vi "io.command-builder.DI.vi"(8 "error in":errorcluster, 11 "IoConf in":T1={"ADDR"=0, "Label"="", "Type"=enum."DI", "Mode"=enum."RIO", "Value"="", "Tags"="", "calibration"=[]} {"calibration"."Y" format="%#.3f"; "calibration"."X" format="%#.3f"; "ADDR" format="%04d"}) -> (0 "error out":errorcluster, 2 "Generated Command":string)   [LabVIEW 2024]
uses:
  controls/IONode.ctl
  controls/type.address.ctl
  controls/enum.io.type.ctl
  controls/enum.io.mode.ctl
  controls/typeXyPoint.ctl
  controls/enum.io-rio.ctl
  variantCtrlNumber.vi
panel:
  in  "Value in":cluster{"value":u8, "timeoutSeconds":u16}
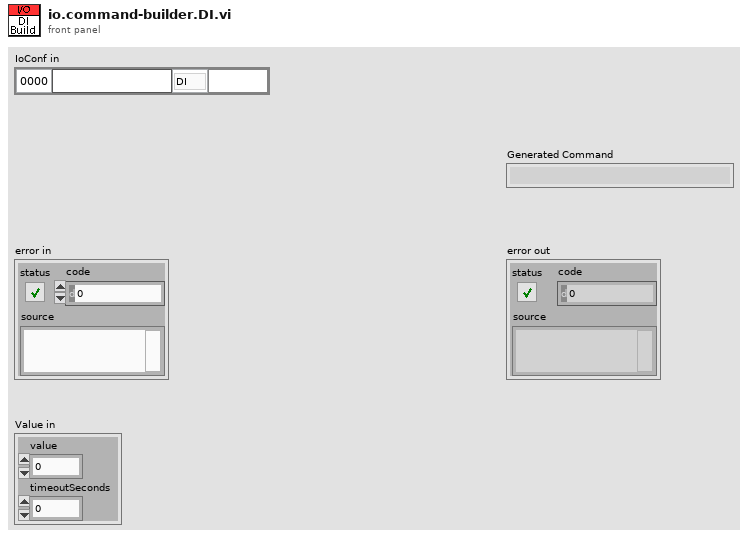
[diagram p1: front panel]
types:
  T1 = typedef "IONode.ctl" = cluster{"ADDR":T2, "Label":string, "Type":T3, "Mode":T4, "Value":string, "Tags":string, "calibration":T5[]}
  T2 = typedef "type.address.ctl" = u16
  T3 = typedef "enum.io.type.ctl" = enum16{"Type", "DI", "DO", "AI", "AO", "VL", "BUF"}
  T4 = typedef "enum.io.mode.ctl" = enum16{"Mode", "RIO", "SIM"}
  T5 = typedef "typeXyPoint.ctl" = cluster{"X":dbl, "Y":dbl}
  T6 = cluster{"DataSize":u8, "Address":u8, "Command(DPORTS)":u8}
  T7 = typedef "enum.io-rio.ctl" = enum16{"RIO_CALIBRATION"}
  T8 = cluster{"WRITE_DO":u8, "Address":T2, "Channel":u8, "value":u8, "timeoutSeconds":u16}
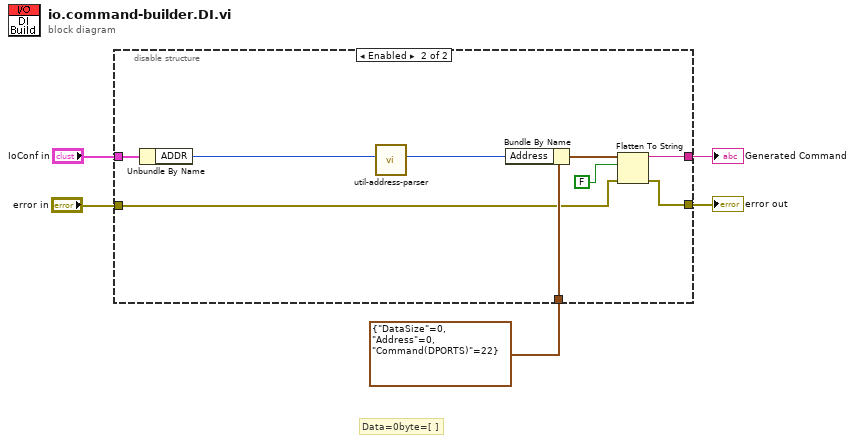
[diagram p0: block diagram]
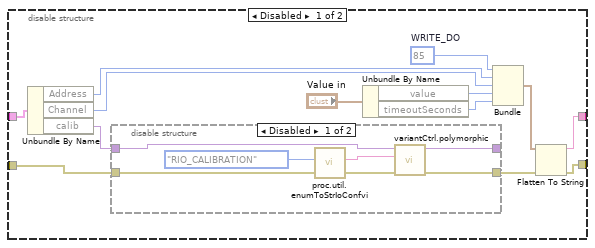
[diagram p2: hidden frame]
diagram:
  # "Data=0byte=[ ]"
  n1 = disable-structure shown="Enabled" {
    disable-tunnel: [w18 w35] -> w5
    disable-tunnel: "IoConf in" -> [w13 w34]
    disable-tunnel: "error in" -> [w11 w30]
    disable-tunnel: [w6 w29] -> w2
    disable-tunnel: T6 {"DataSize"=0, "Address"=0, "Command(DPORTS)"=22} ("output cluster") -> [_ w33]
    frame Disabled {
      w10 = u8 85  # WRITE_DO
      n2 = Unbundle By Name(w13) -> ("Address"=w16:T2, "Channel"=w17:u8, "calib"=w15:variant)
      n3 = disable-structure shown="Disabled" {
        disable-tunnel: w15 -> [w24 w26]
        disable-tunnel: [w23 w26] -> _
        disable-tunnel: [w22 w25] -> w14
        disable-tunnel: w11 -> [w19 w25]
        frame Disabled {
          n4 = call "proc.util.enumToStrIoConfvi.vi"("Step var"=enum.io-rio."RIO_CALIBRATION") -> ("String"=w21:string)  [unwired: 10 in]
          n5 = call-poly "variantCtrl.polymorphic.vi"("error in"=w19, "name in"=w21, "variant in"=w24) -> ("error out"=w22:errorcluster, "variant out"=w23:variant)  [unwired: 5 in, 2 out]
        }
        frame Enabled {
        }
      }
      n6 = Unbundle By Name("Value in") -> ("value"=w9:u8, "timeoutSeconds"=w8:u16)
      n7 = Bundle("WRITE_DO"=w10, "Address"=w16, "Channel"=w17, "value"=w9, "timeoutSeconds"=w8) -> (w7:T8)  [unwired: 1 in]
      n8 = Flatten To String(anything=w7, error in (no error)=w14) -> (data string=w18:string, error out=w6:errorcluster)  [unwired: 2 in, 1 out]
    }
    frame Enabled {
      n9 = Unbundle By Name(w34) -> ("ADDR"=w28:T2)
      n10 = call "util-address-parser.vi"("ADDR 2"=w28) -> ("Address"=w27:u8)  [unwired: 9 in, 1 out]
      n11 = Bundle By Name(cluster=w33, "Address"=w27) -> (w32:T6)
      n12 = Flatten To String(anything=w32, prepend array or string size? (T)=FALSE, error in (no error)=w30) -> (data string=w35:string, error out=w29:errorcluster)  [unwired: 1 in, 1 out]
    }
  }
  "Generated Command" <- w5
  "error out" <- w2
